vi "LocalizeVI.vi"(8 "error in (no error)":errorcluster, 9 "Target Language":string, 10 "Dictionary":T1, 11 "VI in":refnum<vi>) -> (0 "error out":errorcluster)   [LabVIEW 2017, in "JKI Simple Localization.lvlib"]
uses:
  API/JKI Simple Localization.lvlib
  <vilib>/Utility/traverseref.llb/TRef TravTarget.ctl
  <vilib>/Utility/traverseref.llb/VI Scripting - Traverse.lvlib
  Definitions/Private/Font -- Cluster.ctl
  Definitions/Private/Phrase Dictionary Entry -- Cluster.ctl
  Definitions/Dictionary--Cluster.ctl
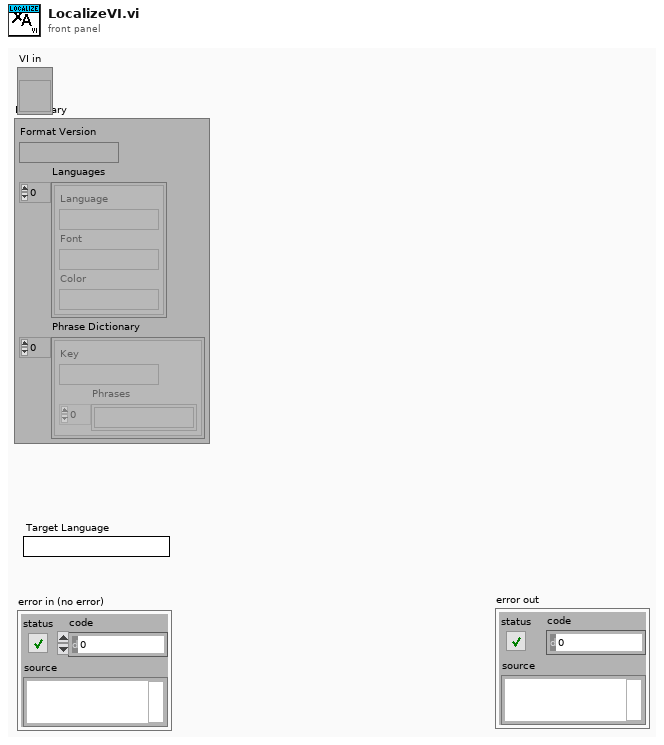
[diagram p1: front panel]
types:
  T1 = typedef "JKI Simple Localization.lvlib/Dictionary--Cluster.ctl" = cluster{"Format Version":string, "Languages":T2[], "Phrase Dictionary":T3[]}
  T2 = typedef "JKI Simple Localization.lvlib/Font -- Cluster.ctl" = cluster{"Language":string, "Font":string, "Color":string}
  T3 = typedef "JKI Simple Localization.lvlib/Phrase Dictionary Entry -- Cluster.ctl" = cluster{"Key":string, "Phrases":string[]}
  T4 = typedef "TRef TravTarget.ctl" = enum16{"FP", "BD", "Other"}
  T5 = typedef "JKI Simple Localization.lvlib/Font Info -- Cluster.ctl" = cluster{"Custom Font Name":bool, "Font Name":string, "Custom Color":bool, "Custom Colorbox":u32}
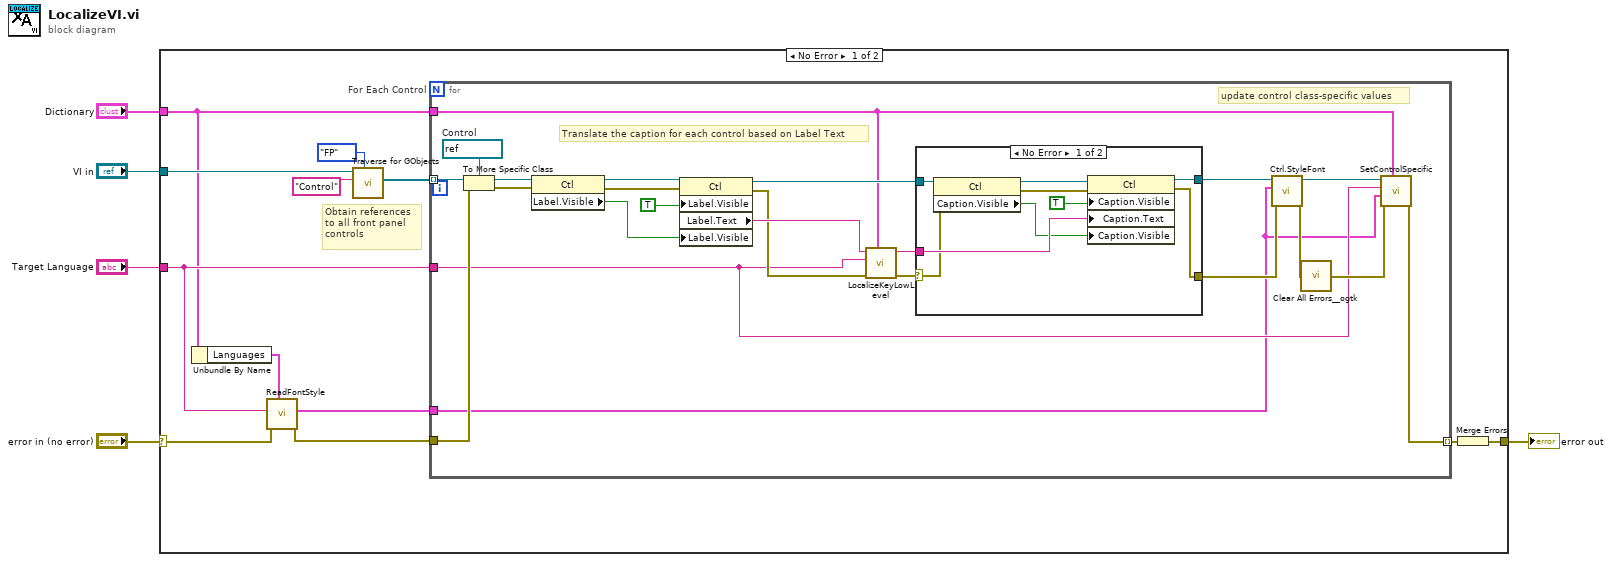
[diagram p0: block diagram]
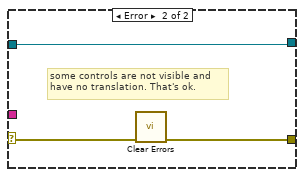
[diagram p2: hidden frame]
diagram:
  n1 = case shown="No Error" "error in (no error)" {
    selector: "error in (no error)" -> [w9 w53]
    tunnel: "VI in" -> [w15 _]
    tunnel: [w12 w53] -> w4
    tunnel: "Dictionary" -> [w7 _]
    tunnel: "Target Language" -> [w10 _]
    frame No Error {
      # "Obtain references to all front panel controls"
      n2 = Unbundle By Name(w7) -> ("Languages"=w6:T2[])
      n3 = call "ReadFontStyle.vi"("Fonts"=w6, "error in (no error)"=w9, "Target Language"=w10) -> ("error out"=w11:errorcluster, "Font Info"=w8:T5)  [unwired: 7 in]
      n4 = call <vilib>:"Traverse for GObjects.vi"("Traverse Target"=TRef_TravTarget."FP", "Class Name"="Control", "VI Refnum"=w15) -> ("References"=w16:refnum<vi>[])  [unwired: 5 in, 3 out]
      n5 = for "For Each Control" {
        tunnel: w16 -> [w40] mode=indexing
        tunnel: w11 -> [w38]
        tunnel: w7 -> [w26]
        tunnel: w10 -> [w23]
        tunnel: [w25] -> w17 mode=indexing
        tunnel: w8 -> [w18]
        w39 = refnum<vi> refnum  # Control
        # "update control class-specific values"
        # "Translate the caption for each control based on Label Text"
        n6 = To More Specific Class(target class=w39, reference=w40, error in=w38) -> (specific class reference=w36:refnum<vi>, error out=w30:errorcluster)
        n7 = property class="Ctl"(reference=w36, error in=w30) -> (reference out=w35:refnum<vi>, error out=w29:errorcluster, "Label.Visible"=w34:bool)
        n8 = property class="Ctl"(reference=w35, error in=w29, "Label.Visible"=TRUE, "Label.Visible"=w34) -> (reference out=w31:refnum<vi>, error out=w28:errorcluster, "Label.Text"=w37:string)
        n9 = call "LocalizeKeyLowLevel.vi"("Dictionary"=w26, "error in (no error)"=w28, "Target Language"=w23, "Key"=w37) -> ("error out"=w27:errorcluster, "Localized Phrase"=w32:string)  [unwired: 6 in]
        n10 = case shown="No Error" w27 {
          selector: w27 -> [w42 w52]
          tunnel: w32 -> [w48 _]
          tunnel: w31 -> [w47 w50]
          tunnel: [w43 w51] -> w20
          tunnel: [w41 w50] -> w22
          frame No Error {
            n11 = property class="Ctl"(reference=w47, error in=w42) -> (reference out=w46:refnum<vi>, error out=w44:errorcluster, "Caption.Visible"=w45:bool)
            n12 = property class="Ctl"(reference=w46, error in=w44, "Caption.Visible"=TRUE, "Caption.Text"=w48, "Caption.Visible"=w45) -> (reference out=w41:refnum<vi>, error out=w43:errorcluster)
          }
          frame Error {
            # "some controls are not visible and \nhave no translation. That's ok."
            n13 = call <vilib>:"Clear Errors.vi"("error in (no error)"=w52) -> ("error out"=w51:errorcluster)  [unwired: 5 in, 1 out]
          }
        }
        n14 = call "Ctrl.StyleFont.vi"("error in (no error)"=w20, "Font Info"=w18, "Ctl Ref in"=w22) -> ("error out"=w19:errorcluster, "Ctl Ref out"=w21:refnum<vi>)  [unwired: 7 in]
        n15 = call <userlib>:"Clear All Errors__ogtk.vi"("Error In"=w19) -> ("Error Out"=w24:errorcluster)  [unwired: 3 in]
        n16 = call "SetControlSpecific.vi"("Dictionary"=w26, "error in (no error)"=w24, "Font Info"=w18, "Target Language"=w23, "Control Reference"=w21) -> ("error out"=w25:errorcluster)  [unwired: 5 in, 1 out]
      }
      n17 = Merge Errors(w17) -> (w12:errorcluster)
    }
    frame Error {
    }
  }
  "error out" <- w4
